vi "Minesweeper-Labview.vi"() -> ()   [LabVIEW 2020]
uses:
  d834ac4b-52eb-48af-9a96-7b33cfe40c1e.vi
  <vilib>/Utility/inputDevices.llb/mouseAcquire.vi
panel:
  out "Mines left":dbl
  out "Array 2":u16[][](array[ring])
  in  "mines":dbl
  in  "height":dbl
  in  "width":dbl
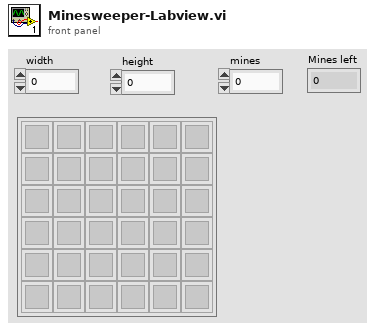
[diagram p1: front panel]
types:
  T1 = typedef "LVRectTypeDef.ctl" = cluster{"Left":i16, "Top":i16, "Right":i16, "Bottom":i16}
  T2 = cluster{"Horizontal":i32, "Vertical":i32, "Scrolling":i32}
  T3 = cluster{"button 1":bool, "button 2":bool, "button 3":bool, "button 4":bool}
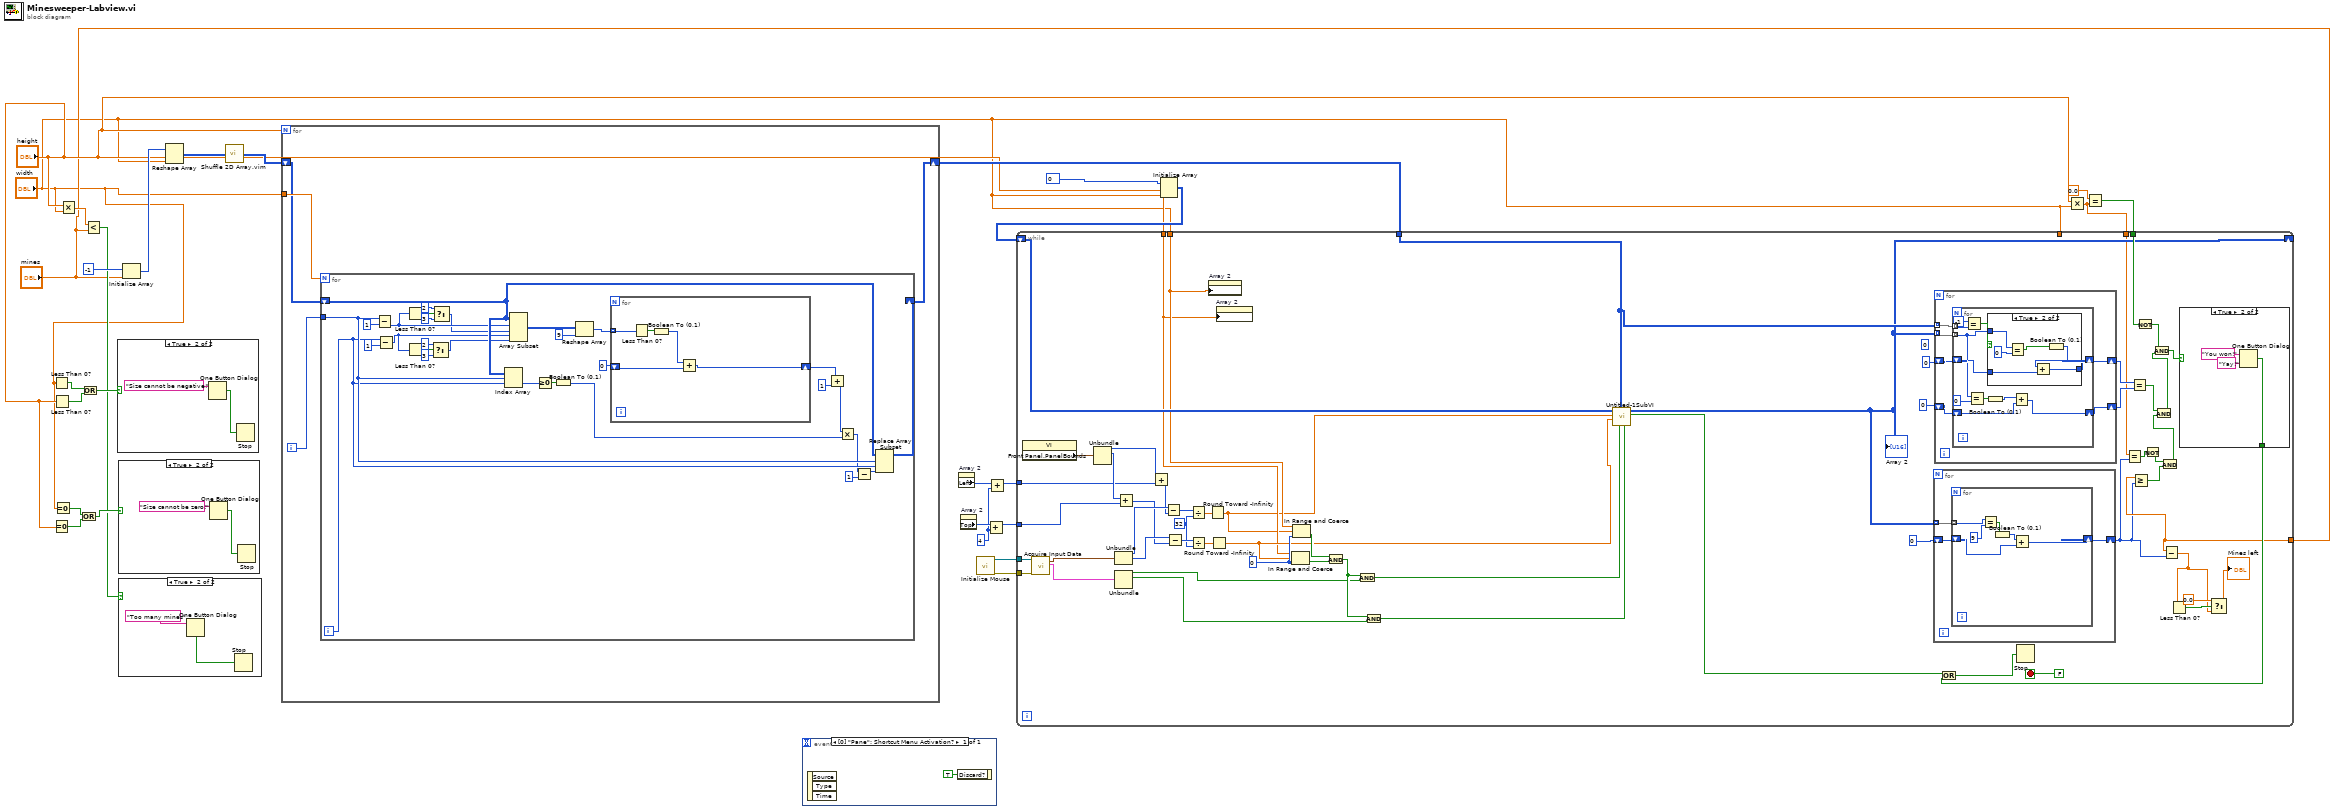
[diagram p0: block diagram]
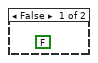
[diagram p3: hidden frame]
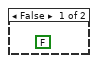
[diagram p4: hidden frame]
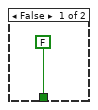
[diagram p5: hidden frame]
diagram:
  w15 = u16 0 items=["", "1", "2", "3", "4", "5", "6", "7", "8", "Flag"]
  w16 = 4
  n1 = Less Than 0?(x="width") -> (x < 0?=w12:bool)
  n2 = Equal To 0?(x="height") -> (x = 0?=w9:bool)
  n3 = Less Than 0?(x="height") -> (x < 0?=w11:bool)
  n4 = Equal To 0?(x="width") -> (x = 0?=w8:bool)
  n5 = Multiply(x="height", y="width") -> (x*y=w25:dbl)
  n6 = Or(x=w8, y=w9) -> (x .or. y?=w10:bool)
  n7 = Or(x=w12, y=w11) -> (x .or. y?=w13:bool)
  n8 = Less?(x=w25, y="mines") -> (x < y?=w7:bool)
  n9 = case shown="True" w13 {
    frame False {
      (unwired) FALSE ("true")
    }
    frame True {
      n10 = One Button Dialog(message="Size cannot be negative!") -> (true=w29:bool)  [unwired: 1 in]
      n11 = Stop(stop? (T)=w29) -> ()
    }
  }
  n12 = case shown="True" w10 {
    frame False {
      (unwired) FALSE ("true")
    }
    frame True {
      n13 = One Button Dialog(message="Size cannot be zero!") -> (true=w31:bool)  [unwired: 1 in]
      n14 = Stop(stop? (T)=w31) -> ()
    }
  }
  n15 = case shown="True" w7 {
    frame False {
    }
    frame True {
      n16 = One Button Dialog(message="Too many mines") -> (true=w34:bool)  [unwired: 1 in]
      n17 = Stop(stop? (T)=w34) -> ()
    }
  }
  n18 = Initialize Array(-1, "mines") -> (w27:i32[])
  n19 = Reshape Array(w27, "height", "width") -> (w26:i32[][])
  n20 = call "Shuffle 2D Array.vim"("array"=w26) -> ("shuffled array"=w24:i32[][])  [unwired: 4 in]
  n21 = for {
    N: "height" -> [_]
    tunnel: "width" -> [w38]
    shift-right: [w35] -> w14
    shift-left: w24 -> [w36]
    i -> [w37]
    n22 = for {
      N: w38 -> [_]
      tunnel: w37 -> [w58]
      shift-right: [w55] -> w35
      shift-left: w36 -> [w59]
      i -> [w57]
      n23 = Subtract(x=w58, y=1) -> (x-y=w48:i32)
      n24 = Subtract(x=w57, y=1) -> (x-y=w40:i32)
      n25 = Less Than 0?(x=w48) -> (x < 0?=w47:bool)
      n26 = Less Than 0?(x=w40) -> (x < 0?=w43:bool)
      n27 = Select(t=2, s=w43, f=3) -> (s? t:f=w39:i32)
      n28 = Select(t=2, s=w47, f=3) -> (s? t:f=w44:i32)
      n29 = Index Array(array=w59, index (row)=w58, index (col)=w57) -> (element=w62:i32)
      n30 = Array Subset(array=w59, index (row)=w48, length (row)=w44, index (col)=w40, length (col)=w39) -> (w50:i32[][])
      n31 = Greater Or Equal To 0?(x=w62) -> (x >= 0?=w63:bool)
      n32 = Boolean To (0,1)(Boolean=w63) -> (0, 1=w60:i16)
      n33 = Reshape Array(w50, 9) -> (w49:i32[])
      n34 = for {
        tunnel: w49 -> [w72] mode=indexing
        shift-right: [w68] -> w61
        shift-left: 0 -> [w71]
        n35 = Less Than 0?(x=w72) -> (x < 0?=w70:bool)
        n36 = Boolean To (0,1)(Boolean=w70) -> (0, 1=w69:i16)
        n37 = Add(x=w69, y=w71) -> (x+y=w68:i32)
      }
      n38 = Add(x=w61, y=1) -> (x+y=w52:i32)
      n39 = Multiply(x=w52, y=w60) -> (x*y=w56:i32)
      n40 = Subtract(x=w56, y=1) -> (x-y=w54:i32)
      n41 = Replace Array Subset(array=w59, new element=w54, index (row)=w58, index (col)=w57) -> (w55:i32[][])
    }
  }
  n42 = event shown="[0] \"Pane\": Shortcut Menu Activation?" {
    selector: _ -> [_]
    dyn-events: _ -> [_]
    timeout: _ -> [_]
    event Shortcut Menu Activation? {
      n43 = event-data() -> ()  [unwired: 1 in, 3 out]
      n44 = event-data("Discard?"=TRUE) -> ()  [unwired: 1 in, 1 out]
    }
  }
  n45 = property on="Array 2" class="Arr (strict)"() -> ("Left"=w19:i32)  [unwired: 2 in, 2 out]
  n46 = property on="Array 2" class="Arr (strict)"() -> ("Top"=w20:i32)  [unwired: 2 in, 2 out]
  n47 = call <vilib>:"Initialize Mouse.vi"() -> ("error out"=w22:errorcluster, "device ID"=w23:refnum<k1>)  [unwired: 10 in]
  n48 = Add(x=w20, y=w16) -> (x+y=w17:i32)
  n49 = Add(x=w19, y=w16) -> (x+y=w18:i32)
  n50 = Initialize Array(w15, "height", "width") -> (w21:u16[][])
  n51 = Multiply(x="height", y="width") -> (x*y=w1:dbl)
  n52 = Equal?(x=0.0, y=w1) -> (x = y?=w5:bool)
  n53 = while {
    tunnel: w23 -> [w131]
    tunnel: w22 -> [w130]
    tunnel: "width" -> [w92]
    tunnel: "height" -> [w91]
    tunnel: w14 -> [w96]
    shift-right: [w90] -> _
    shift-left: w21 -> [w109]
    tunnel: w17 -> [w108]
    tunnel: w18 -> [w107]
    tunnel: w5 -> [w97]
    tunnel: "mines" -> [w82]
    tunnel: "width" -> [_]
    tunnel: w1 -> [w80]
    stop <- FALSE stop-if-true
    (unwired) u16 0
    w116 = 0
    w119 = 32
    n54 = property class="VI"() -> ("Front Panel.PanelBounds"=w106:T1)  [unwired: 2 in, 2 out]
    n55 = call-poly <vilib>:"Acquire Input Data.vi"("device ID"=w131, "error in (no error)"=w130) -> ("axis info"=w128:T2, "button info"=w129:T3)  [unwired: 14 in, 2 out]
    n56 = Unbundle(w106) -> ("Left"=w123:i16, "Top"=w122:i16)  [unwired: 2 out]
    n57 = Unbundle(w128) -> ("Horizontal"=w127:i32, "Vertical"=w126:i32)  [unwired: 1 out]
    n58 = Unbundle(w129) -> ("button 1"=w112:bool, "button 2"=w111:bool)  [unwired: 2 out]
    n59 = Add(x=w122, y=w108) -> (x+y=w124:i32)
    n60 = Add(x=w123, y=w107) -> (x+y=w125:i32)
    n61 = Subtract(x=w127, y=w125) -> (x-y=w121:i32)
    n62 = Subtract(x=w126, y=w124) -> (x-y=w120:i32)
    n63 = Divide(x=w121, y=w119) -> (x/y=w118:dbl)
    n64 = Divide(x=w120, y=w119) -> (x/y=w117:dbl)
    n65 = property on="Array 2" class="Arr (strict)"("Number of Columns"=w92) -> ()  [unwired: 2 in, 2 out]
    n66 = Round Toward -Infinity(1:w118) -> (0:w75:dbl)
    n67 = Round Toward -Infinity(1:w117) -> (0:w104:dbl)
    n68 = property on="Array 2" class="Arr (strict)"("Number of Rows"=w91) -> ()  [unwired: 2 in, 2 out]
    n69 = In Range and Coerce(upper limit=w91, x=w104, lower limit=w116) -> (In Range?=w114:bool)  [unwired: 1 out]
    n70 = In Range and Coerce(upper limit=w92, x=w75, lower limit=w116) -> (In Range?=w115:bool)  [unwired: 1 out]
    n71 = And(x=w115, y=w114) -> (x .and. y?=w113:bool)
    n72 = And(x=w113, y=w112) -> (x .and. y?=w110:bool)
    n73 = And(x=w113, y=w111) -> (x .and. y?=w105:bool)
    n74 = call "Untitled-1SubVI.vi"("Boolean"=w105, "Boolean 2"=w110, "shuffled array"=w96, "Numeric"=w104, "Numeric 2"=w75, "Array in"=w109) -> ("true"=w74:bool, "Array out"=w90:u16[][])  [unwired: 4 in]
    "Array 2" <- w90
    n75 = for {
      shift-right: [w134] -> w81
      shift-left: u16 0 ("y") -> [w133]
      tunnel: w90 -> [w132] mode=indexing
      n76 = for {
        shift-right: [w138] -> w134
        shift-left: w133 -> [w137]
        tunnel: w132 -> [w140] mode=indexing
        n77 = Equal?(x=w140, y=u16 9) -> (x = y?=w135:bool)
        n78 = Boolean To (0,1)(Boolean=w135) -> (0, 1=w136:i16)
        n79 = Add(x=w136, y=w137) -> (x+y=w138:u16)
      }
    }
    n80 = for {
      tunnel: w90 -> [w150] mode=indexing
      shift-right: [w149] -> w94
      shift-left: 0 -> [w148]
      tunnel: w96 -> [w147] mode=indexing
      shift-right: [w146] -> w93
      shift-left: i16 0 -> [w145]
      n81 = for {
        tunnel: w150 -> [w156] mode=indexing
        shift-right: [w157] -> w149
        shift-left: w148 -> [w158]
        tunnel: w147 -> [w161] mode=indexing
        shift-right: [w152] -> w146
        shift-left: w145 -> [w151]
        n82 = Equal?(x=-1, y=w161) -> (x = y?=w159:bool)
        n83 = Equal?(x=w156, y=u16 0) -> (x = y?=w153:bool)
        n84 = Boolean To (0,1)(Boolean=w153) -> (0, 1=w154:i16)
        n85 = case shown="True" w159 {
          tunnel: w156 -> [_ w168]
          tunnel: w158 -> [w162 w165]
          tunnel: [w162 w164] -> w157
          frame False {
          }
          frame True {
            n86 = Equal?(x=w168, y=u16 0) -> (x = y?=w163:bool)
            n87 = Boolean To (0,1)(Boolean=w163) -> (0, 1=w166:i16)
            n88 = Add(x=w166, y=w165) -> (x+y=w164:i32)
          }
        }
        n89 = Add(x=w154, y=w151) -> (x+y=w152:i16)
      }
    }
    n90 = Equal?(x=w80, y=w81) -> (x = y?=w79:bool)
    n91 = Equal?(x=w94, y=w93) -> (x = y?=w84:bool)
    n92 = Greater Or Equal?(x=w82, y=w81) -> (x >= y?=w76:bool)
    n93 = Not(x=w97) -> (.not. x?=w98:bool)
    n94 = Not(x=w79) -> (.not. x?=w78:bool)
    n95 = And(x=w78, y=w76) -> (x .and. y?=w77:bool)
    n96 = And(x=w84, y=w77) -> (x .and. y?=w83:bool)
    n97 = And(x=w98, y=w83) -> (x .and. y?=w99:bool)
    n98 = Subtract(x=w82, y=w81) -> (x-y=w86:dbl)
    n99 = Less Than 0?(x=w86) -> (x < 0?=w88:bool)
    n100 = case shown="True" w99 {
      tunnel: [FALSE ("true") w143] -> w102
      frame False {
      }
      frame True {
        n101 = One Button Dialog(message="You won!", button name ("OK")="Yay!") -> (true=w143:bool)
      }
    }
    n102 = Or(x=w74, y=w102) -> (x .or. y?=w101:bool)
    n103 = Stop(stop? (T)=w101) -> ()
    n104 = Select(t=0.0, s=w88, f=w86) -> (s? t:f=→"Mines left":dbl)
  }
